vi "TC Simulation Data.vi"(4 "Function":T2(ring), 5 "error in (no error)":errorcluster, 7 "Machine Name":T1, 8 "State In":enum16{"Off", "On"}(ring)) -> (0 "error out":errorcluster, 2 "Cooler State":enum16{"Off", "On"}(ring), 3 "Fan State":enum16{"Off", "On"}(ring))   [LabVIEW 2020, in "Startup Processes.lvlib"]
doc: "This VI stores the DAQ setup parameters. This is the type of signal, physical channel, scaling information and filtering options"
uses:
  Startup Processes.lvlib
  _typedefs/Subpanel Names.ctl
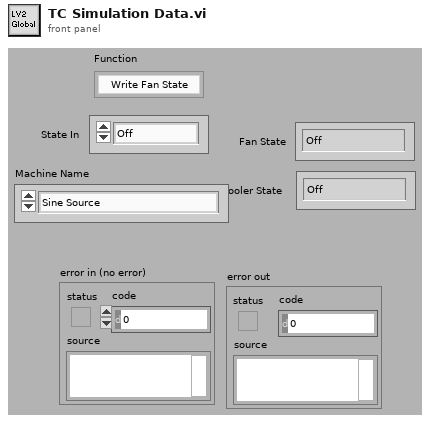
[diagram p1: front panel]
types:
  T1 = typedef "Startup Processes.lvlib/Subpanel Names.ctl" = enum16{"Sine Source", "Ramp Source", "Hen House TC", "Dog House TC", "Out House TC"}
  T2 = enum16{"Write Fan State", "Write Cooler State", "Read"}
  T3 = cluster{"Fan State":enum16{"Off", "On"}, "Cooler State":enum16{"Off", "On"}}
  T4 = cluster{"Fan State":enum16{"Off", "On"}, "Cooler State":enum16{"Off", "On"}}[]
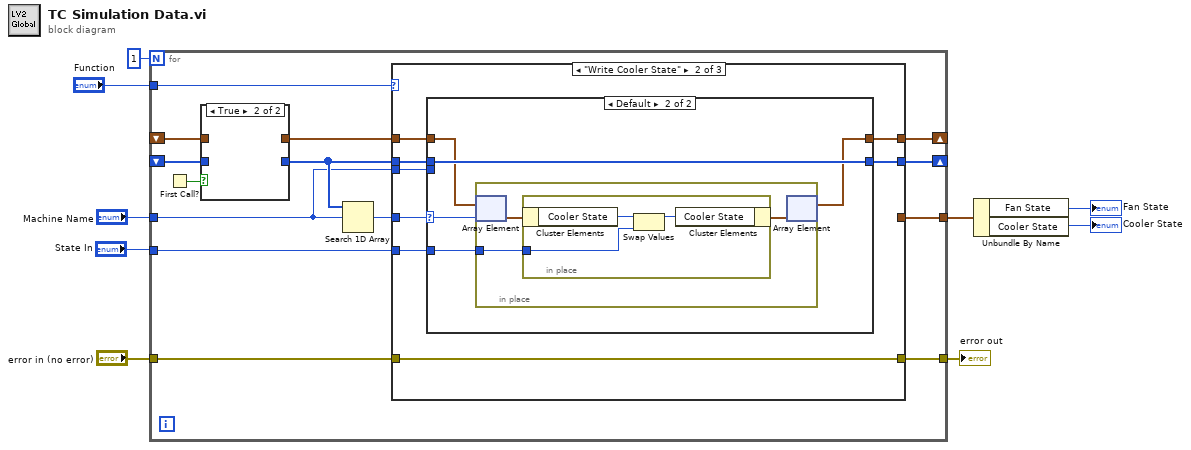
[diagram p0: block diagram]
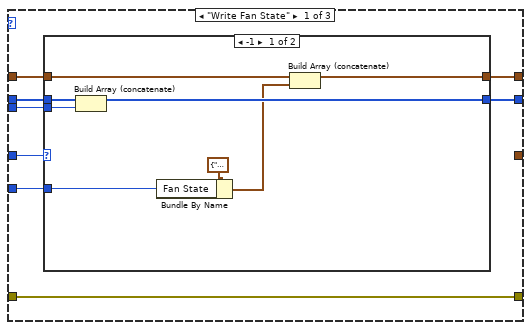
[diagram p3: hidden frame]
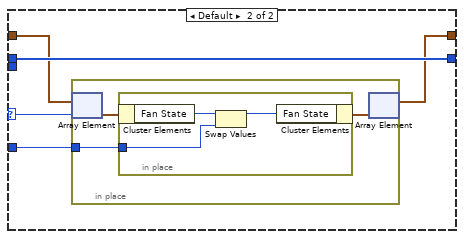
[diagram p4: hidden frame]
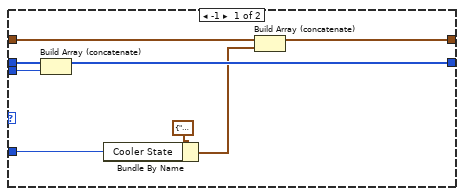
[diagram p5: hidden frame]
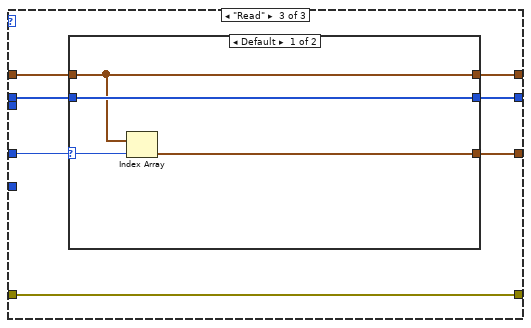
[diagram p6: hidden frame]
diagram:
  n1 = for {
    N: 1 -> [_]
    tunnel: "Function" -> [w23]
    shift-right: [w21] -> _
    shift-left: _ -> [w16]
    tunnel: "State In" -> [w22]
    tunnel: [w20] -> w8
    tunnel: "error in (no error)" -> [w19]
    shift-right: [w14] -> _
    shift-left: _ -> [w15]
    tunnel: "Machine Name" -> [w11]
    tunnel: [w10] -> w1
    n2 = First Call?() -> (First Call?: T/F=w18:bool)
    n3 = case shown="True" w18 {
      tunnel: [w25 _] -> w17
      tunnel: w16 -> [w25 _]
      tunnel: w15 -> [w24 _]
      tunnel: [w24 _] -> w13
      frame False {
      }
      frame True {
      }
    }
    n4 = Search 1D Array(1D array=w13, element=w11) -> (index of element=w12:i32)  [unwired: 1 in]
    n5 = case shown="\"Write Cooler State\"" w23 {
      tunnel: [w31 w54 w82] -> w21
      tunnel: w17 -> [w32 w59 w85]
      tunnel: w22 -> [w30 w55 _]
      tunnel: [w33 w60 w86] -> w20
      tunnel: w19 -> [w33 w60 w86]
      tunnel: [w27 w53 w81] -> w14
      tunnel: w13 -> [w28 w58 w84]
      tunnel: w12 -> [w29 w56 w83]
      tunnel: w11 -> [w26 w57 _]
      tunnel: [_ _ w80] -> w10
      frame "Write Fan State" {
        n6 = case shown="-1" w29 {
          selector: w29 -> [_ w44]
          tunnel: w32 -> [w35 w45]
          tunnel: [w34 w42] -> w31
          tunnel: w30 -> [w37 w43]
          tunnel: w28 -> [w41 w46]
          tunnel: [w39 w46] -> w27
          tunnel: w26 -> [w40 _]
          frame -1 {
            n7 = Build Array (concatenate)(w41, w40) -> (w39:T1[])
            n8 = Bundle By Name(cluster=T3 {"Fan State"=enum."Off", "Cooler State"=enum."Off"}, "Fan State"=w37) -> (w36:T3)
            n9 = Build Array (concatenate)(w35, w36) -> (w34:T4)
          }
          frame Default {
            n10 = in-place {
              in-place-border: w43 -> [w48]
              n11 = in-place-array #1(w45, w44) -> (w49:T3)
              n12 = in-place {
                in-place-border: w48 -> [w50]
                n13 = in-place-cluster #2(w49) -> ("Fan State"=w52:enum16{"Off", "On"})
                n14 = Swap Values(12:w52, 14:w50) -> (1:w51:enum16{"Off", "On"})  [unwired: 1 in, 1 out]
                n15 = in-place-cluster #2("Fan State"=w51) -> (w47:T3)
              }
              n16 = in-place-array #1(w47) -> (w42:T4)  [unwired: 1 out]
            }
          }
        }
      }
      frame "Write Cooler State" {
        n17 = case shown="Default" w56 {
          selector: w56 -> [_ w71]
          tunnel: w59 -> [w62 w72]
          tunnel: [w61 w69] -> w54
          tunnel: w55 -> [w64 w70]
          tunnel: w58 -> [w68 w73]
          tunnel: [w66 w73] -> w53
          tunnel: w57 -> [w67 _]
          frame -1 {
            n18 = Build Array (concatenate)(w68, w67) -> (w66:T1[])
            n19 = Bundle By Name(cluster=T3 {"Fan State"=enum."Off", "Cooler State"=enum."Off"}, "Cooler State"=w64) -> (w63:T3)
            n20 = Build Array (concatenate)(w62, w63) -> (w61:T4)
          }
          frame Default {
            n21 = in-place {
              in-place-border: w70 -> [w75]
              n22 = in-place-array #3(w72, w71) -> (w76:T3)
              n23 = in-place {
                in-place-border: w75 -> [w77]
                n24 = in-place-cluster #4(w76) -> ("Cooler State"=w79:enum16{"Off", "On"})
                n25 = Swap Values(12:w79, 14:w77) -> (1:w78:enum16{"Off", "On"})  [unwired: 1 in, 1 out]
                n26 = in-place-cluster #4("Cooler State"=w78) -> (w74:T3)
              }
              n27 = in-place-array #3(w74) -> (w69:T4)  [unwired: 1 out]
            }
          }
        }
      }
      frame "Read" {
        n28 = case shown="Default" w83 {
          selector: w83 -> [w89 _]
          tunnel: w85 -> [w88 w92]
          tunnel: w84 -> [w90 w91]
          tunnel: [w88 w92] -> w82
          tunnel: [w90 w91] -> w81
          tunnel: [w87 _] -> w80
          frame Default {
            n29 = Index Array(array=w88, index=w89) -> (element=w87:T3)
          }
          frame -1 {
          }
        }
      }
    }
  }
  "error out" <- w8
  n30 = Unbundle By Name(w1) -> ("Fan State"=→"Fan State":enum16{"Off", "On"}, "Cooler State"=→"Cooler State":enum16{"Off", "On"})
